vi "DAQ.Read AI and Write AO.vi"(8 "error in (no error)":errorcluster, 11 "Instrument.DAQ in":refnum<class "Instrument.DAQ.lvclass">) -> (0 "error out":errorcluster, 3 "Instrument.DAQ out":refnum<class "Instrument.DAQ.lvclass">)   [LabVIEW 2019, in "Instrument.Lockin.lvlib" / "Instrument.DAQ.lvclass"]
uses:
  Instrument.DAQ.lvclass
  DAQmx/DAQmx.lvclass
  C:/Program Files/National Instruments/LabVIEW 2019/vi.lib/JKI/JKI SMO/SMO/SMO.lvclass
panel:
  in  "Display Data":bool
  out "Diagnostic Graph":dbl[][](graph)
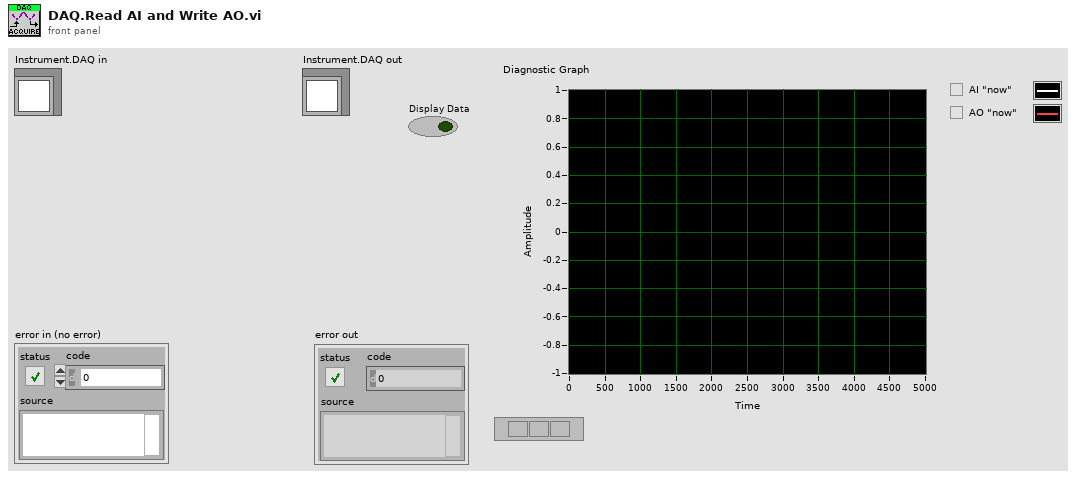
[diagram p1: front panel]
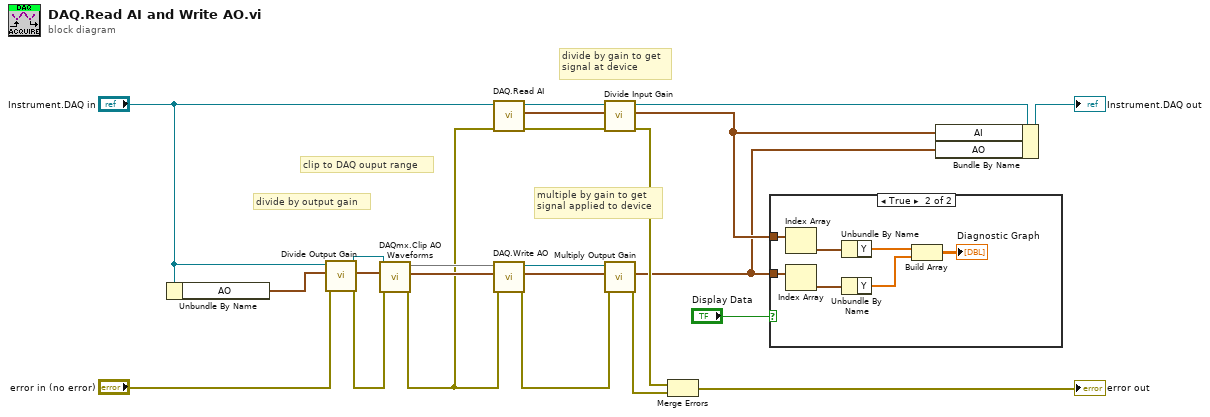
[diagram p0: block diagram]
diagram:
  # "divide by gain to get\nsignal at device"
  # "multiple by gain to get\nsignal applied to device"
  # "clip to DAQ ouput range"
  # "divide by output gain"
  n1 = Unbundle By Name("Instrument.DAQ in") -> ("AO"=w3:waveform(dbl)[])
  n2 = call "Divide Output Gain.vi"("error in (no error)"="error in (no error)", "WFM in"=w3, "Instrument.DAQ"="Instrument.DAQ in") -> ("error out"=w20:errorcluster, "WFM out"=w22:waveform(dbl)[], "Instrument.DAQ out"=w21:refnum<class "Instrument.DAQ.lvclass">)  [unwired: 6 in]
  n3 = call "DAQmx.Clip AO Waveforms.vi"("error in (no error)"=w20, "AO []"=w22, 11:w21) -> ("error out"=w10:errorcluster, "Clipped AO []"=w11:waveform(dbl)[], 3:w19)  [unwired: 6 in]
  n4 = call "DAQ.Read AI.vi"("error in"=w10, "Instrument.DAQ in"="Instrument.DAQ in") -> ("error out"=w15:errorcluster, "AI []"=w17:waveform(dbl)[], "Instrument.DAQ out"=w16:refnum<class "Instrument.DAQ.lvclass">)  [unwired: 6 in, 1 out]
  n5 = call "DAQ.Write AO.vi"("error in (no error)"=w10, "AO []"=w11, "Instrument.DAQ in"=w19) -> ("error out"=w14:errorcluster, "AO out []"=w13:waveform(dbl)[], "Instrument.DAQ out"=w18:refnum<class "Instrument.DAQ.lvclass">)  [unwired: 6 in]
  n6 = call "Divide Input Gain.vi"("error in (no error)"=w15, "WFM in"=w17, "Instrument.DAQ"=w16) -> ("error out"=w12:errorcluster, "WFM out"=w5:waveform(dbl)[], "Instrument.DAQ out"=w7:refnum<class "Instrument.DAQ.lvclass">)  [unwired: 6 in]
  n7 = call "Multiply Output Gain.vi"("error in (no error)"=w14, "WFM in"=w13, "Instrument.DAQ"=w18) -> ("error out"=w8:errorcluster, "WFM out"=w4:waveform(dbl)[])  [unwired: 6 in, 1 out]
  n8 = Merge Errors(w12, w8) -> (→"error out":errorcluster)
  n9 = case shown="True" "Display Data" {
    tunnel: w5 -> [_ w25]
    tunnel: w4 -> [_ w24]
    frame False {
    }
    frame True {
      n10 = Index Array(array=w25) -> (element=w30:waveform(dbl))  [unwired: 1 in]
      n11 = Index Array(array=w24) -> (element=w28:waveform(dbl))  [unwired: 1 in]
      n12 = Unbundle By Name(w30) -> ("Y"=w29:dbl[])
      n13 = Unbundle By Name(w28) -> ("Y"=w27:dbl[])
      n14 = Build Array(w29, w27) -> (→"Diagnostic Graph":dbl[][])
    }
  }
  n15 = Bundle By Name(cluster=w7, "AI"=w5, "AO"=w4) -> (→"Instrument.DAQ out":refnum<class "Instrument.DAQ.lvclass">)
